vi "format_answer.vi"(10 "answer string":string) -> (0 "crc":u8, 1 "switches":bool[](array[boolean]), 2 "address":u8, 3 "return command":u8, 4 "answer as byte array":u8[](array[numeric]))   [LabVIEW 2018]
doc: "formats the string that holds the answer of a command"
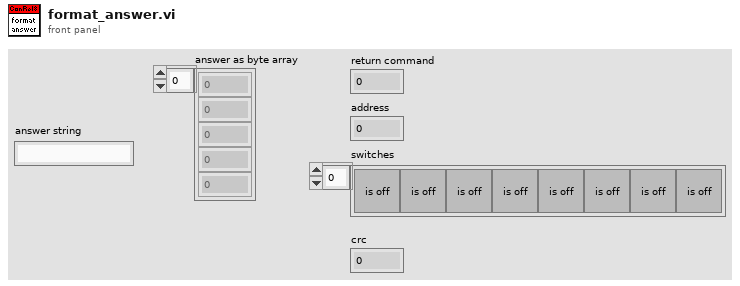
[diagram p1: front panel]
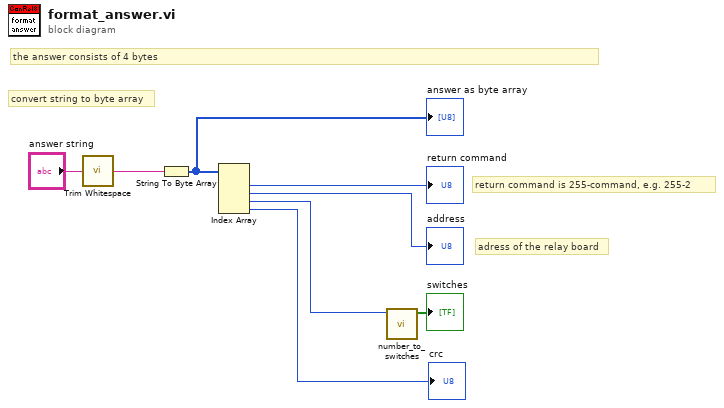
[diagram p0: block diagram]
diagram:
  # "adress of the relay board"
  # "return command is 255-command, e.g. 255-2"
  # "the answer consists of 4 bytes"
  # "convert string to byte array"
  n1 = call <vilib>:"Trim Whitespace.vi"("string"="answer string") -> ("trimmed string"=w7:string)  [unwired: 1 in]
  n2 = String To Byte Array(string=w7) -> (unsigned byte array=w6:u8[])
  "answer as byte array" <- w6
  n3 = Index Array(array=w6) -> (element #1=→"return command":u8, element #2=→"address":u8, element #3=w3:u8, element #4=→"crc":u8)  [unwired: 4 in]
  n4 = call "number_to_switches.vi"("number"=w3) -> ("switches"=→"switches":bool[])  [unwired: 5 in, 1 out]
